vi "camera_acquisition_continously.vi"(0 "Detektionskamera":T1="cam0", 1 "BufferInterval":u32, 2 "Video Mode":u32=2, 3 "Shutter time (ms)":dbl=100.0) -> (4 "Kamera eingeschaltet?":bool, 5 "Detektionskamera":T1 caption="Session Out", 6 "Image Memory":T2, 7 "Ereignis: FrameDone?":refnum<event-registration>, 8 "error out":errorcluster)   [LabVIEW 2009]
uses:
  <vilib>/userDefined/High Color/IMAQdx.ctl
  <vilib>/vision/Image Controls.llb/IMAQ Image.ctl
  <vilib>/vision/driver/IMAQdx.llb/IMAQdx Acquisition Mode.ctl
  <vilib>/vision/driver/NI_Vision_Acquisition_Software.lvlib
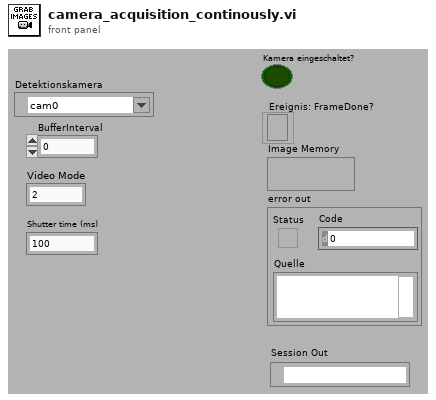
[diagram p1: front panel]
types:
  T1 = typedef "IMAQdx.ctl" = refnum<k21>
  T2 = typedef "IMAQ Image.ctl" = refnum<image>
  T3 = typedef "Image Type" = u32
  T4 = typedef "NI_Vision_Acquisition_Software.lvlib/IMAQdx Acquisition Mode.ctl" = enum32{"One Shot", "Continuous"}
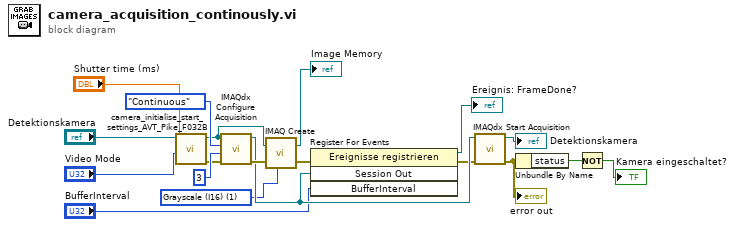
[diagram p0: block diagram]
diagram:
  w3 = T3 1 items=["Grayscale (U8)", "Grayscale (I16)", "Grayscale (SGL)", "Complex (CSG)", "RGB (U32)", "HSL (U32)", "RGB (U64)", "Grayscale (U16)"] ("Image Type")
  n1 = call "camera_initialise_start_settings_AVT_Pike_F032B.vi"("Video Mode"="Video Mode", "Shutter time (ms)"="Shutter time (ms)", "Camera In"="Detektionskamera") -> ("Fehler (Ausgang)"=w12:errorcluster, "Camera Out"=w13:T1)  [unwired: 7 in]
  n2 = call <vilib>:"IMAQdx Configure Acquisition.vi"("error in"=w12, "Number of Buffers"=u32 3, "Continuous?"=IMAQdx_Acquisition_Mode."Continuous", "Session In"=w13) -> ("error out"=w14:errorcluster, "Session Out"=w11:T1)  [unwired: 6 out]
  n3 = call "IMAQ Create"("Image Name"=w13, "Image Type"=w3, "error in (no error)"=w14) -> ("New Image"=→"Image Memory":T2, "error out"=w15:errorcluster)  [unwired: 1 in, 1 out]
  n4 = register-events(error in=w15, w11, "BufferInterval") -> (reference out=→"Ereignis: FrameDone?":refnum<event-registration>, error out=w10:errorcluster)  [unwired: 1 in]
  n5 = call <vilib>:"IMAQdx Start Acquisition.vi"("error in"=w10, "Session In"=w11) -> ("error out"=w16:errorcluster, "Session Out"=→"Detektionskamera":T1)  [unwired: 8 out]
  "error out" <- w16
  n6 = Unbundle By Name(w16) -> ("status"=w17:bool)
  n7 = Not(x=w17) -> (.not. x?=→"Kamera eingeschaltet?":bool)
